vi "Read Glimpse One Frame.vi"(5 "#frame to read (1,2,...,end)":i32, 6 "Header file data":T1 {"Pixel depth" items=["8 bits", "16 bits", "Float", "Complex", "RGB", "HSL"]; "time of 1st frame, \nsec since 1/1/04" format="%.2f"}, 7 "Data Folder":path) -> (2 "wait time of certain frame (ms)":u32, 3 "Image":T5(plugin-control))   [LabVIEW 2014]
uses:
  4.Other/header ctl/Header file data.ctl
  4.Other/header ctl/Offset table.ctl
  4.Other/header ctl/Offset.ctl
  4.Other/header ctl/file number.ctl
panel:
  out "TTB Array (ms)\ntime axis (ms)":u32[](array[numeric])
  out "wait time between each frame (ms)":u32[](array[numeric])
  out "Width":i32=1200
  out "Height":i32=1920
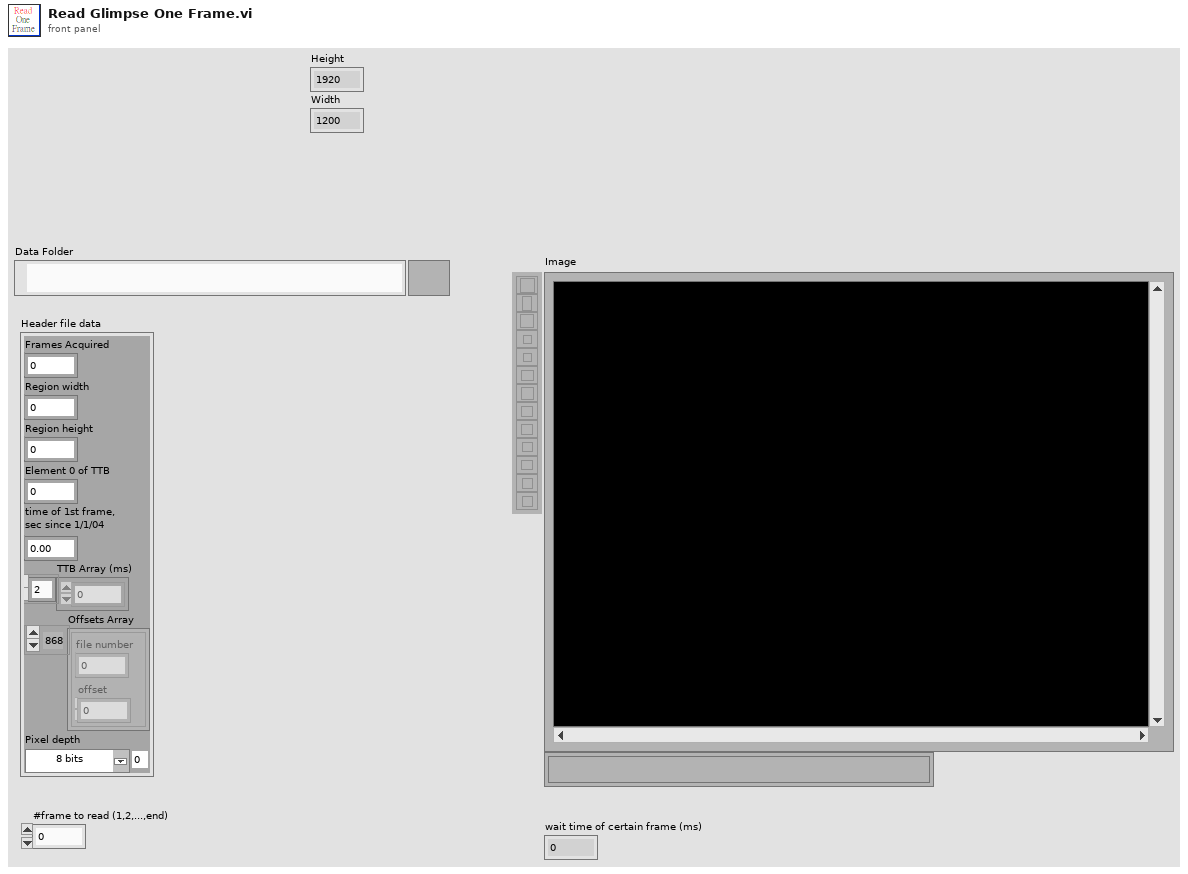
[diagram p1: front panel]
types:
  T1 = typedef "Header file data.ctl" = cluster{"Frames Acquired":u32, "Region width":i32, "Region height":i32, "Element 0 of TTB":u32, "time of 1st frame, \nsec since 1/1/04":dbl, "TTB Array (ms)":u32[], "Offsets Array":T2, "Pixel depth":u32}
  T2 = typedef "Offset table.ctl" = cluster{"offset":T3, "file number":T4}[]
  T3 = typedef "Offset.ctl" = i32
  T4 = typedef "file number.ctl" = u8
  T5 = typedef "IMAQ Image.ctl" = refnum<image>
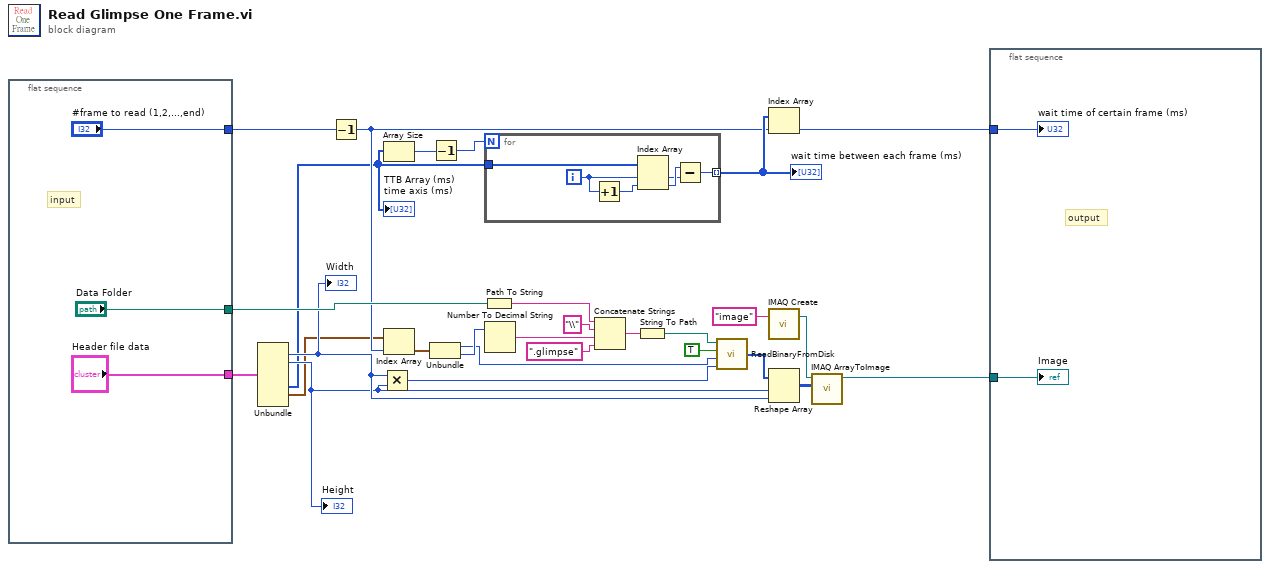
[diagram p0: block diagram]
diagram:
  n1 = flat-sequence {
    tunnel: ["Data Folder"] -> w28
    tunnel: ["#frame to read (1,2,...,end)"] -> w21
    tunnel: ["Header file data"] -> w5
    frame #0 {
      # "input"
    }
  }
  n2 = Unbundle(w5) -> ("Region width"=w4:i32, "Region height"=w3:i32, "TTB Array (ms)"=w2:u32[], "Offsets Array"=w1:T2)  [unwired: 4 out]
  "Height" <- w3
  "Width" <- w4
  "TTB Array (ms)\ntime axis (ms)" <- w2
  n3 = Decrement(x=w21) -> (x-1=w7:i32)
  n4 = Multiply(x=w4, y=w3) -> (x*y=w27:i32)
  n5 = Array Size(array=w2) -> (size(s)=w23:i32)
  n6 = Index Array(array=w1, index=w7) -> (element=w9:cluster{"offset":T3, "file number":T4})
  n7 = Unbundle(w9) -> ("offset"=w11:T3, "file number"=w18:T4)
  n8 = Decrement(x=w23) -> (x-1=w22:i32)
  n9 = Path To String(path=w28) -> (string=w26:string)
  n10 = for {
    N: w22 -> [_]
    tunnel: w2 -> [w37]
    tunnel: [w32] -> w8 mode=indexing
    i -> [w36]
    n11 = Increment(x=w36) -> (x+1=w35:i32)
    n12 = Index Array(array=w37, index #1=w36, index #2=w35) -> (element #1=w33:u32, element #2=w34:u32)
    n13 = Subtract(x=w34, y=w33) -> (x-y=w32:u32)
  }
  "wait time between each frame (ms)" <- w8
  n14 = Number To Decimal String(number=w18) -> (decimal integer string=w17:string)  [unwired: 1 in]
  n15 = Concatenate Strings(w26, "\\" ("string"), w17, ".glimpse" ("string")) -> (w15:string)
  n16 = String To Path(string=w15) -> (path=w10:path)
  n17 = call "ReadBinaryFromDisk.vi"("size to read (count)"=w27, "offset (in bytes) (0)"=w11, "Set Position?"=TRUE, "Read or Write Path"=w10) -> ("data (U8)"=w14:u8[])  [unwired: 1 in, 1 out]
  n18 = Index Array(array=w8, index=w7) -> (element=w6:u32)
  n19 = call "IMAQ Create"("Image Name"="image") -> ("New Image"=w24:T5)  [unwired: 4 in, 1 out]
  n20 = Reshape Array(w14, w3, w4) -> (w13:u8[][])
  n21 = call "IMAQ ArrayToImage"("Image Pixels (U8)"=w13, "Image"=w24) -> ("Image Out"=w12:T5)  [unwired: 8 in, 1 out]
  n22 = flat-sequence {
    tunnel: w12 -> [w39]
    tunnel: w6 -> [w38]
    frame #0 {
      # "output"
      "Image" <- w39
      "wait time of certain frame (ms)" <- w38
    }
  }
